vi "read_txt_parameters.vi"(0 "Loading mode":T2(ring), 1 "Output format":T1(ring), 5 "file name":string, 7 "pid":string, 11 "error in":errorcluster) -> (4 "String Array output":string[][](array[string]), 6 "Double Array output":dbl[][](array[numeric]) format="%0.3f", 8 "Decimal Array Output":i64[][](array[numeric]), 10 "Single string output":string, 15 "error out":errorcluster)   [LabVIEW 2010]
uses:
  <vilib>/Utility/file.llb/Read From Spreadsheet File (string).vi
  <vilib>/Utility/file.llb/Read From Spreadsheet File (DBL).vi
  <vilib>/Utility/file.llb/Read From Spreadsheet File (I64).vi
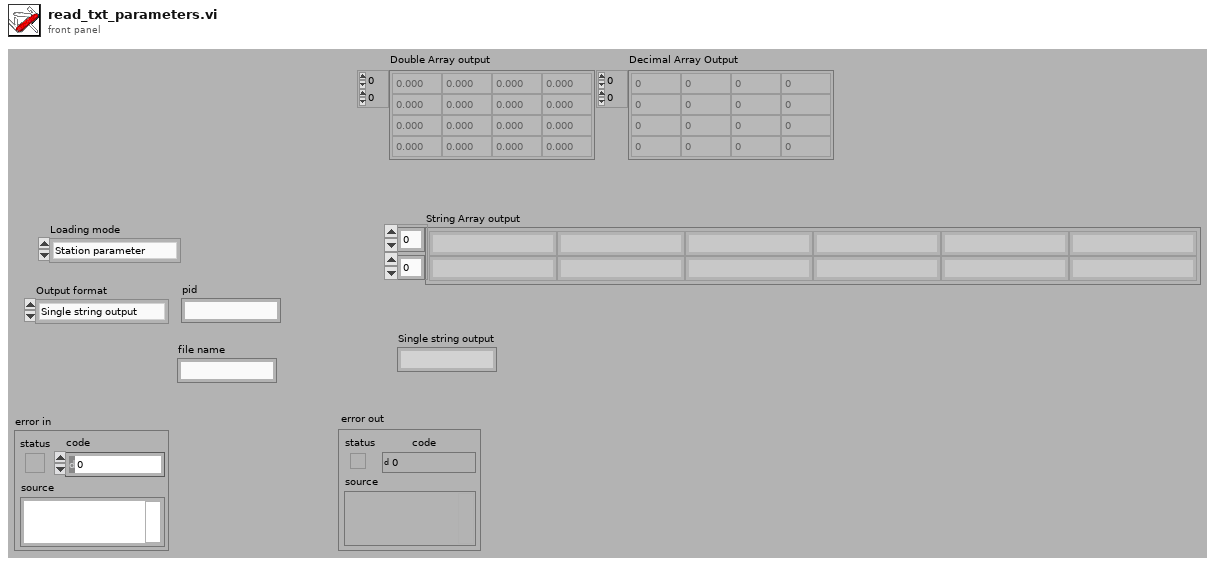
[diagram p1: front panel]
types:
  T1 = enum16{"Single string output", "String Array ouput", "Double Array output", "Decimal Array output"}
  T2 = enum16{"Station parameter", "Product definition", "AOA validation step parameter", "pm2 step parameter", "AOA station cal step parameter", "Station cal Step parameter", "Global variables"}
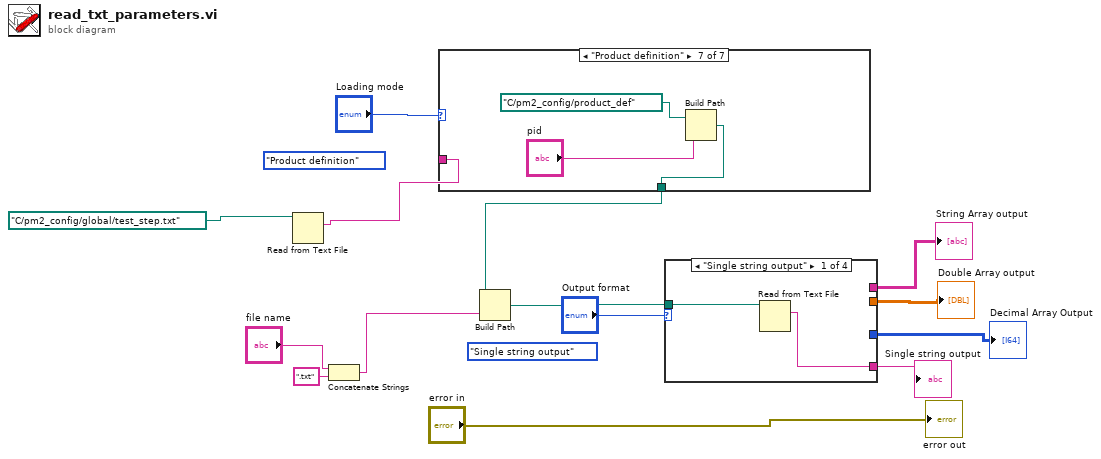
[diagram p0: block diagram]
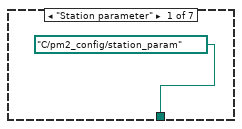
[diagram p2: hidden frame]
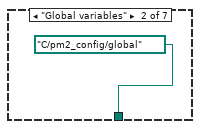
[diagram p3: hidden frame]
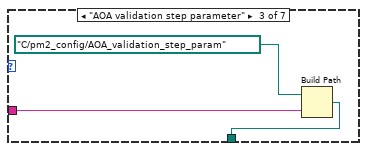
[diagram p4: hidden frame]
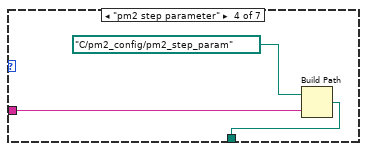
[diagram p5: hidden frame]
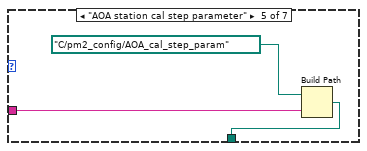
[diagram p6: hidden frame]
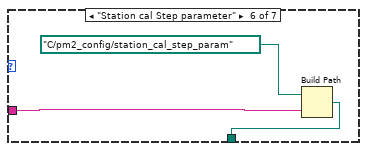
[diagram p7: hidden frame]
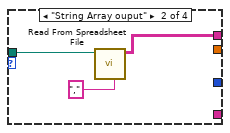
[diagram p8: hidden frame]
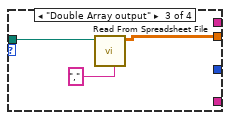
[diagram p9: hidden frame]
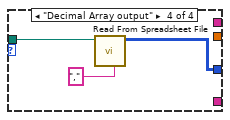
[diagram p10: hidden frame]
diagram:
  (unwired) T1."Single string output"
  (unwired) T2."Product definition"
  n1 = Read from Text File(file (use dialog)=path "C:/pm2_config/global/test_step.txt") -> (text=w1:string)  [unwired: 3 in, 3 out]
  n2 = Concatenate Strings("file name", ".txt" ("string")) -> (w14:string)
  n3 = case shown="\"Product definition\"" "Loading mode" {
    tunnel: [path "C:/pm2_config/station_param" ("base path") path "C:/pm2_config/global" ("base path") w18 w21 w24 w27 w29] -> w8
    tunnel: w1 -> [_ _ w17 w20 w23 w26 _]
    frame "Station parameter" {
    }
    frame "Global variables" {
    }
    frame "AOA validation step parameter" {
      n4 = Build Path(base path=path "C:/pm2_config/AOA_validation_step_param", name or relative path=w17) -> (appended path=w18:path)
    }
    frame "pm2 step parameter" {
      n5 = Build Path(base path=path "C:/pm2_config/pm2_step_param", name or relative path=w20) -> (appended path=w21:path)
    }
    frame "AOA station cal step parameter" {
      n6 = Build Path(base path=path "C:/pm2_config/AOA_cal_step_param", name or relative path=w23) -> (appended path=w24:path)
    }
    frame "Station cal Step parameter" {
      n7 = Build Path(base path=path "C:/pm2_config/station_cal_step_param", name or relative path=w26) -> (appended path=w27:path)
    }
    frame "Product definition" {
      n8 = Build Path(base path=path "C:/pm2_config/product_def", name or relative path="pid") -> (appended path=w29:path)
    }
  }
  n9 = Build Path(base path=w8, name or relative path=w14) -> (appended path=w10:path)
  n10 = case shown="\"Single string output\"" "Output format" {
    tunnel: w10 -> [w33 w36 w39 w42]
    tunnel: [w32 _ _ _] -> w9
    tunnel: [_ w35 _ _] -> w7
    tunnel: [_ _ w37 _] -> w5
    tunnel: [_ _ _ w40] -> w4
    frame "Single string output" {
      n11 = Read from Text File(file (use dialog)=w33) -> (text=w32:string)  [unwired: 3 in, 3 out]
    }
    frame "String Array ouput" {
      n12 = call-poly <vilib>:"Read From Spreadsheet File.vi"("delimiter (\\t)"="," ("delimiter (\\t)"), "file path (dialog if empty)"=w36) -> ("all rows"=w35:string[][])  [unwired: 5 in, 4 out]
    }
    frame "Double Array output" {
      n13 = call-poly <vilib>:"Read From Spreadsheet File.vi"("delimiter (\\t)"="," ("delimiter (\\t)"), "file path (dialog if empty)"=w39) -> ("all rows"=w37:dbl[][])  [unwired: 5 in, 4 out]
    }
    frame "Decimal Array output" {
      n14 = call-poly <vilib>:"Read From Spreadsheet File.vi"("delimiter (\\t)"="," ("delimiter (\\t)"), "file path (dialog if empty)"=w42) -> ("all rows"=w40:i64[][])  [unwired: 5 in, 4 out]
    }
  }
  "String Array output" <- w7
  "Single string output" <- w9
  "Double Array output" <- w5
  "Decimal Array Output" <- w4
  "error out" <- "error in"
